vi "S2C_Shared_Proc_ReportError.vi"(8 "Error In":errorcluster) -> (0 "Error Out":errorcluster)   [LabVIEW 2024]
uses:
  Globals/S2C_Globals.vi
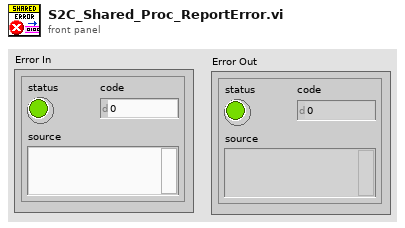
[diagram p1: front panel]
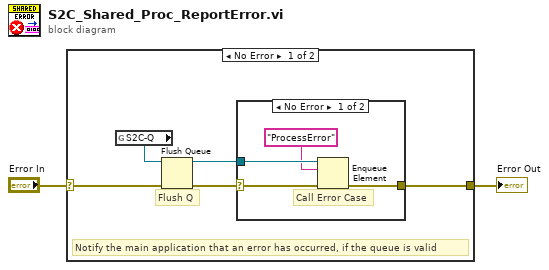
[diagram p0: block diagram]
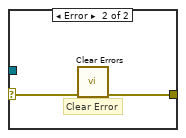
[diagram p2: hidden frame]
diagram:
  n1 = case shown="No Error" "Error In" {
    selector: "Error In" -> [w4 w14]
    tunnel: [w5 w14] -> w2
    frame No Error {
      # "Notify the main application that an error has occurred, if the queue is valid"
      # "Flush Q"
      n2 = global read "S2C_Globals.vi" "S2C-Q"() -> (w7:refnum<queue>)
      n3 = Flush Queue(queue=w7, error in (no error)=w4) -> (queue out=w6:refnum<queue>, error out=w3:errorcluster)  [unwired: 1 out]
      n4 = case shown="No Error" w3 {
        selector: w3 -> [w8 w13]
        tunnel: w6 -> [w11 _]
        tunnel: [w9 w12] -> w5
        frame No Error {
          # "Call Error Case"
          n5 = Enqueue Element(queue=w11, element="ProcessError", error in (no error)=w8) -> (error out=w9:errorcluster)  [unwired: 1 in, 2 out]
        }
        frame Error {
          # "Clear Error"
          n6 = call <vilib>:"Clear Errors.vi"("error in (no error)"=w13) -> ("error out"=w12:errorcluster)  [unwired: 5 in, 1 out]
        }
      }
    }
    frame Error {
    }
  }
  "Error Out" <- w2
